vi "CST_EVM Plugin pointers.vi"() -> (0 "Pointers":T1)   [LabVIEW 2010, in "lib1299.lvlib"]
uses:
  lib1299.lvlib
  TYP_EVM Plugin Pointers.ctl
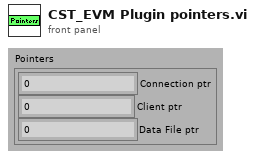
[diagram p1: front panel]
types:
  T1 = typedef "lib1299.lvlib/TYP_EVM Plugin Pointers.ctl" = cluster{"Connection ptr":u32, "Client ptr":u32, "Data File ptr":u32}
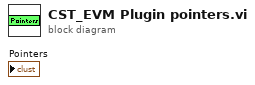
[diagram p0: block diagram]
diagram:
